vi "(33) part 2 que.vi"() -> ()   [LabVIEW 2025]
uses:
  <vilib>/numeric/Random Number (Range) U64.vi
  <vilib>/numeric/sub_Random U32.vi
panel:
  in  "stop":bool
  out "Waveform Chart":dbl(graph)
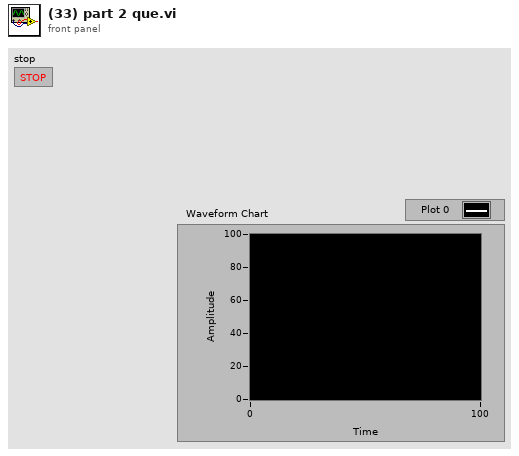
[diagram p1: front panel]
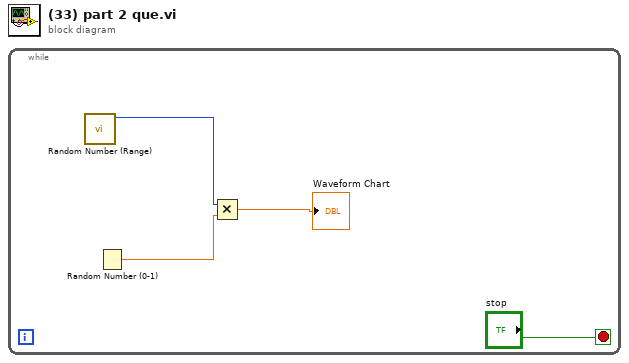
[diagram p0: block diagram]
diagram:
  n1 = while {
    stop <- "stop" stop-if-true
    n2 = call-poly <vilib>:"Random Number (Range).vi"() -> ("number"=w4:u64)  [unwired: 11 in]
    n3 = Random Number (0-1)() -> (number: 0 to 1=w3:dbl)
    n4 = Multiply(x=w4, y=w3) -> (x*y=→"Waveform Chart":dbl)
  }
